vi "up arrow.vi"() -> (3 "^":u8)   [LabVIEW 2025, in "AOC.lvlib"]
uses:
  AOC.lvlib
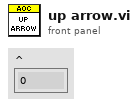
[diagram p1: front panel]
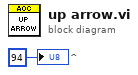
[diagram p0: block diagram]
diagram:
  "^" <- u8 94 ("element")
